vi "Trigger Laser.vi"(4 "Trigger Pin":u8, 5 "Laser Pin":u8, 6 "error in (no error)":errorcluster, 7 "milliseconds to wait":u32, 8 "DI Value in":bool, 9 "LINX Resource in":T1) -> (0 "error out":errorcluster, 2 "DI Value out":bool, 3 "LINX Resource out":T1)   [LabVIEW 2022 SP3]
uses:
  <vilib>/MakerHub/LINX/Private/Type Defs/LINX Ref.ctl
  <vilib>/MakerHub/LINX/Private/Type Defs/Platform.ctl
  <vilib>/MakerHub/LINX/Private/Type Defs/Interface.ctl
  <vilib>/MakerHub/LINX/Private/Device/Type Defs/LINX Device Config.ctl
  <vilib>/MakerHub/LINX/Private/Device/Type Defs/TCP Config.ctl
  <vilib>/MakerHub/LINX/Private/Device/Type Defs/Channels.ctl
  <vilib>/MakerHub/LINX/Public/Peripherals/PWM/PWM Set Duty Cycle 1 Chan.vi
  <vilib>/MakerHub/LINX/Public/Peripherals/Digital/Digital Read 1 Chan.vi
  <vilib>/MakerHub/LINX/Public/Peripherals/Digital/Digital Read N Chans.vi
  <vilib>/MakerHub/LINX/Private/Local IO/LinxDigitalRead.vi
  <vilib>/MakerHub/LINX/Public/Utilities/Check Channel.vi
  <vilib>/MakerHub/LINX/Public/Peripherals/PWM/PWM Set Duty Cycle N Chans.vi
  <vilib>/MakerHub/LINX/Private/Utilties/Generate Error.vi
  <vilib>/MakerHub/LINX/LMH-LINX.lvlib
  <vilib>/MakerHub/LINX/Private/Device/Device.lvlib
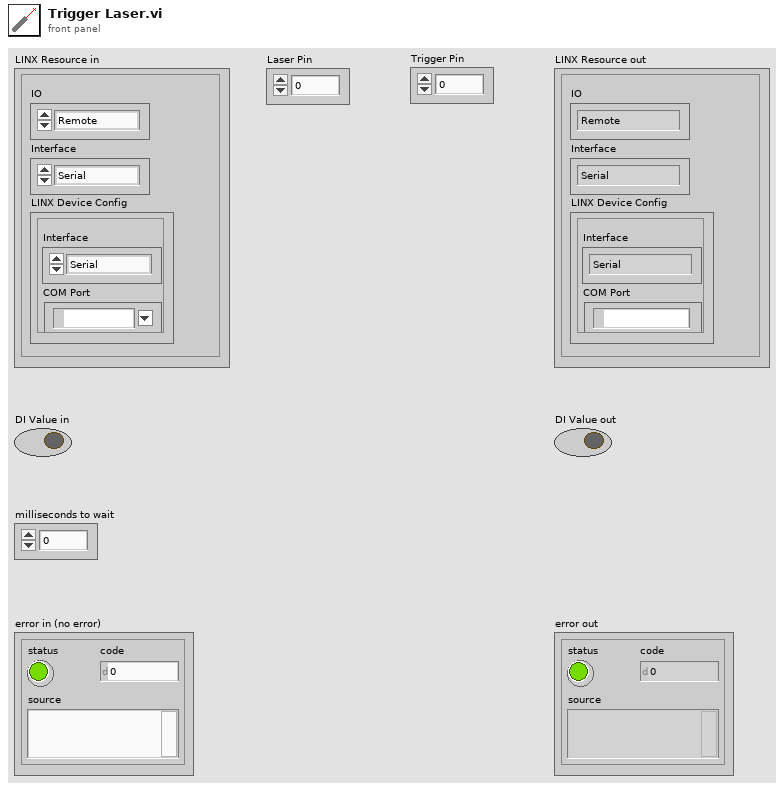
[diagram p1: front panel]
types:
  T1 = typedef "LMH-LINX.lvlib/LINX Ref.ctl" = cluster{"IO":T2, "Interface":T3, "LINX Device Config":T4}
  T2 = typedef "LMH-LINX.lvlib/Platform.ctl" = enum16{"Remote", "Local"}
  T3 = typedef "LMH-LINX.lvlib/Interface.ctl" = enum16{"Serial", "TCP"}
  T4 = typedef "LMH-LINX.lvlib/Device.lvlib/LINX Device Config.ctl" = cluster{"Interface":T3, "COM Port":refnum<visa-resource-name>, "TCP Configuration":T5, "Device Family":u8, "Device ID":u8, "Device Name":string, "TCP Ref":refnum<k5>, "Channels":T6}
  T5 = typedef "LMH-LINX.lvlib/Device.lvlib/TCP Config.ctl" = cluster{"IP Address":string, "Port":u16}
  T6 = typedef "LMH-LINX.lvlib/Channels.ctl" = cluster{"DI":u8[], "DO":u8[], "AI":u8[], "AO":u8[], "PWM":u8[], "QE":u8[], "UART":u8[], "I2C 2":u8[], "SPI":u8[], "CAN":u8[], "Servo":u8[], "AI Ref (V)":dbl, "AI Resolution (Bits)":u8, "AO Ref (V)":dbl, "AO Resolution (Bits)":u8}
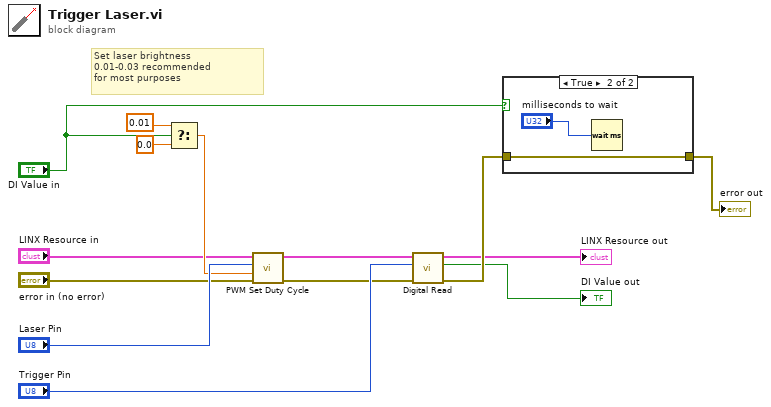
[diagram p0: block diagram]
diagram:
  # "Set laser brightness\n0.01-0.03 recommended\nfor most purposes"
  n1 = Select(t=0.01, s="DI Value in", f=0.0) -> (s? t:f=w10:dbl)
  n2 = call-poly <vilib>:"PWM Set Duty Cycle.vi"("Error In"="error in (no error)", "Duty Cycle (0-1)"=w10, "PWM Channel"="Laser Pin", "LINX Resource"="LINX Resource in") -> ("Error Out"=w5:errorcluster, "LINX Resource"=w2:T1)  [unwired: 6 in]
  n3 = call-poly <vilib>:"Digital Read.vi"("Error In"=w5, "DI Channel"="Trigger Pin", "LINX Resource"=w2) -> ("Error Out"=w8:errorcluster, "DI Value"=→"DI Value out":bool, "LINX Resource"=→"LINX Resource out":T1)  [unwired: 6 in]
  n4 = case shown="True" "DI Value in" {
    tunnel: w8 -> [w15 w16]
    tunnel: [w15 w16] -> w9
    frame False {
    }
    frame True {
      n5 = Wait (ms)(milliseconds to wait="milliseconds to wait") -> ()  [unwired: 1 out]
    }
  }
  "error out" <- w9
